vi "Close.vi"(8 "error in":errorcluster, 11 "Device in":refnum<class "Device.lvclass">) -> (0 "error out":errorcluster, 3 "Device out":refnum<class "Device.lvclass">)   [LabVIEW 2023, in "Device.lvclass"]
uses:
  Device.lvclass
  Device.lvclass/Device.ctl
  Capabilities.lvclass
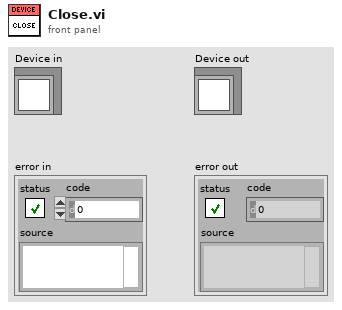
[diagram p1: front panel]
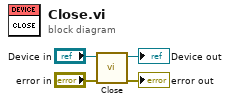
[diagram p0: block diagram]
diagram:
  n1 = call-parent "Close.vi"("error in"="error in", "Capabilities in"="Device in") -> ("error out"=→"error out":errorcluster, "Capabilities out"=→"Device out":refnum<class "Device.lvclass">)  [unwired: 8 in]
